vi "_fgv_sessions.vi"(7 "Operation":T7=enum."GetData", 8 "error in":errorcluster caption="error in (no error)", 10 "Session User Data in (None)":T1={"IDN string"="", "Instrument FW"="", "Instr type"="", "Instr type for err. msg."="", "Installed Options"=[], "Ignore Error Messages"="", "Logging params"=variant, "OPC Timeout"=5000, "VISA Timeout"=10000, "STB Poll VISA Timeout"=5000, "Additional Flags"=4, "Wait Before Read"=0, "Wait Before Write"=0, "Option String Flags"=0, "IO Segment Size"=10000000, "VISA Access Mode"=4, "Interface Type"=enum."TCPIP", "OPC Wait Mode"=enum."STBpolling", "Bin Float Number  Format"=enum."Float_4_Bytes_Swapped", "Bin Integer Number Format"=enum."Int32_4_Bytes_Swapped", "Simulate"=FALSE, "VXIcapable"=TRUE, "Duplicate Session"=FALSE, "Add LF to Write"=TRUE, "Logging"=FALSE, "Fast Sweep"=FALSE, "Query Instrument Status"=TRUE, "Check Range"=TRUE, "Check Options"=TRUE} {"VISA Access Mode" items=["VISA Defaults"=0, "Exclusive Lock"=1, "Load Settings"=4]; "IO Segment Size" format="%#.6p"; "Additional Flags" format="%011b"}, 11 "VISA resource name":refnum<visa-resource-name>) -> (0 "error out":errorcluster, 1 "Session Ix out":i32, 2 "Session User Data out":T1={"IDN string"="", "Instrument FW"="", "Instr type"="", "Instr type for err. msg."="", "Installed Options"=[], "Ignore Error Messages"="", "Logging params"=variant, "OPC Timeout"=5000, "VISA Timeout"=10000, "STB Poll VISA Timeout"=5000, "Additional Flags"=4, "Wait Before Read"=0, "Wait Before Write"=0, "Option String Flags"=0, "IO Segment Size"=10000000, "VISA Access Mode"=4, "Interface Type"=enum."TCPIP", "OPC Wait Mode"=enum."STBpolling", "Bin Float Number  Format"=enum."Float_4_Bytes_Swapped", "Bin Integer Number Format"=enum."Int32_4_Bytes_Swapped", "Simulate"=FALSE, "VXIcapable"=TRUE, "Duplicate Session"=FALSE, "Add LF to Write"=TRUE, "Logging"=FALSE, "Fast Sweep"=FALSE, "Query Instrument Status"=TRUE, "Check Range"=TRUE, "Check Options"=TRUE} {"VISA Access Mode" items=["VISA Defaults"=0, "Exclusive Lock"=1, "Load Settings"=4]; "IO Segment Size" format="%#.6p"; "Additional Flags" format="%011b"}, 3 "VISA resource name out":refnum<visa-resource-name>)   [LabVIEW 2022 SP3, in "hmp4000_rsidr_core.lvlib"]
uses:
  hmp4000_rsidr_core.lvlib
  _type_Operation_Fgv_Session.ctl
  type_Session_Data.ctl
  type_VisaAccessMode.ctl
  type_InterfaceType.ctl
  type_OPC_Wait_Mode.ctl
  type_Binary_Float_Number_Format.ctl
  type_Binary_Integer_Number_Format.ctl
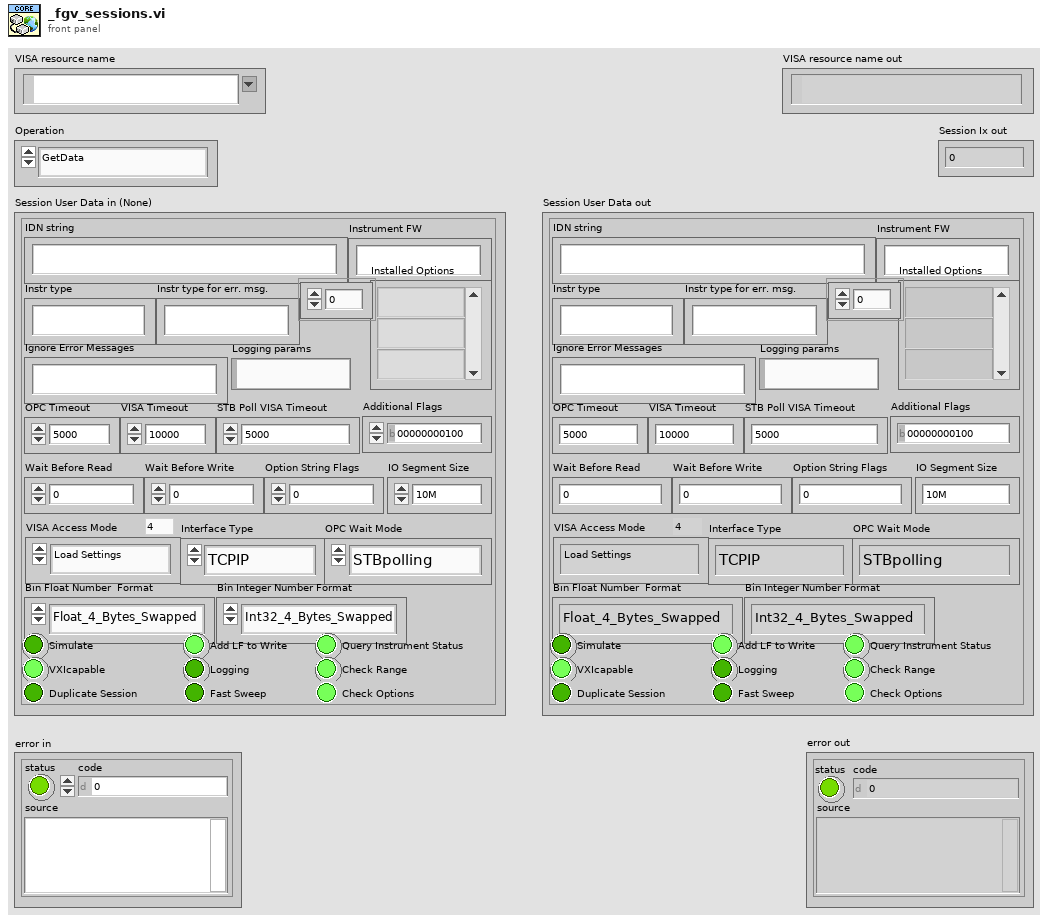
[diagram p1: front panel]
types:
  T1 = typedef "hmp4000_rsidr_core.lvlib/type_Session_Data.ctl" = cluster{"IDN string":string, "Instrument FW":string, "Instr type":string, "Instr type for err. msg.":string, "Installed Options":string[], "Ignore Error Messages":string, "Logging params":variant, "OPC Timeout":i32, "VISA Timeout":i32, "STB Poll VISA Timeout":i32, "Additional Flags":i32, "Wait Before Read":i32, "Wait Before Write":i32, "Option String Flags":i32, "IO Segment Size":i64, "VISA Access Mode":T2, "Interface Type":T3, "OPC Wait Mode":T4, "Bin Float Number  Format":T5, "Bin Integer Number Format":T6, "Simulate":bool, "VXIcapable":bool, "Duplicate Session":bool, "Add LF to Write":bool, "Logging":bool, "Fast Sweep":bool, "Query Instrument Status":bool, "Check Range":bool, "Check Options":bool}
  T2 = typedef "hmp4000_rsidr_core.lvlib/type_VisaAccessMode.ctl" = u16
  T3 = typedef "hmp4000_rsidr_core.lvlib/type_InterfaceType.ctl" = enum16{"Unknown", "GPIB", "VXI", "GPIB_VXI", "ASRL", "PXI", "TCPIP", "USB", "SOCKET"}
  T4 = typedef "hmp4000_rsidr_core.lvlib/type_OPC_Wait_Mode.ctl" = enum16{"STBpolling", "STBpollingSlow", "STBpollingSuperSlow", "ServiceRequest", "OPCquery"}
  T5 = typedef "hmp4000_rsidr_core.lvlib/type_Binary_Float_Number_Format.ctl" = enum16{"Float_4_Bytes_Swapped", "Float_4_Bytes", "Double_8_Bytes_Swapped", "Double_8_Bytes"}
  T6 = typedef "hmp4000_rsidr_core.lvlib/type_Binary_Integer_Number_Format.ctl" = enum16{"Int32_4_Bytes_Swapped", "Int32_4 Bytes", "Int16_2_Bytes_Swapped", "Int16_2_Bytes"}
  T7 = typedef "hmp4000_rsidr_core.lvlib/_type_Operation_Fgv_Session.ctl" = enum16{"Initialize", "GetData", "SetData", "Clear", "GetSessionIx"}
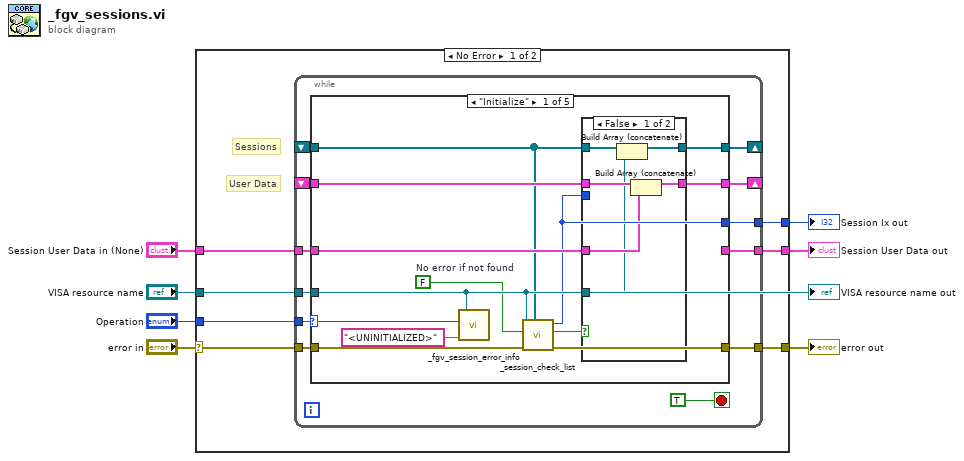
[diagram p0: block diagram]
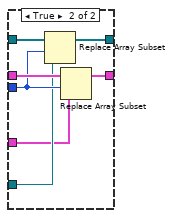
[diagram p2: hidden frame]
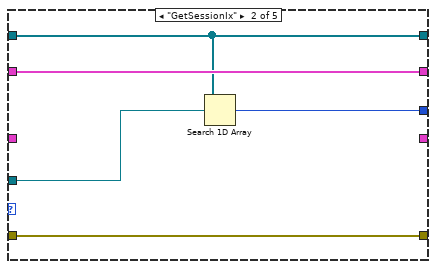
[diagram p3: hidden frame]
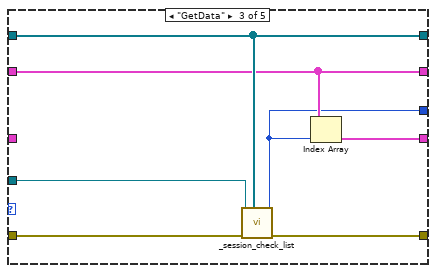
[diagram p4: hidden frame]
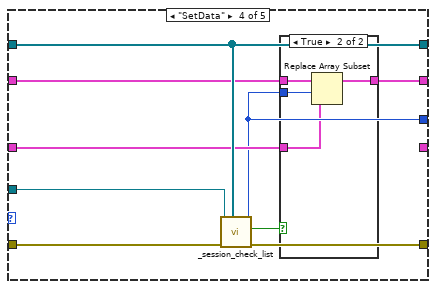
[diagram p5: hidden frame]
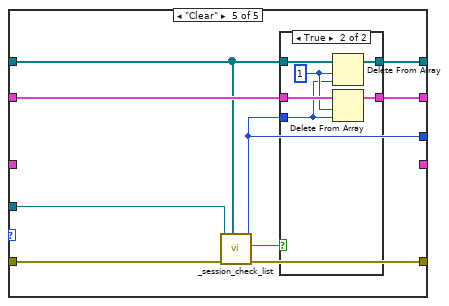
[diagram p7: hidden frame]
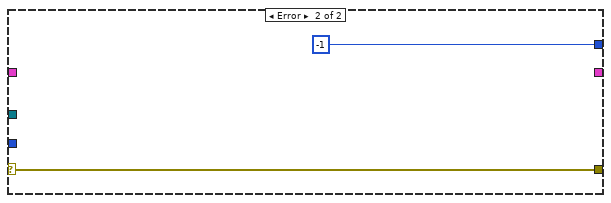
[diagram p9: hidden frame]
diagram:
  n1 = case shown="No Error" "error in" {
    selector: "error in" -> [w13 w97]
    tunnel: "Operation" -> [w10 _]
    tunnel: "Session User Data in (None)" -> [w11 _]
    tunnel: "VISA resource name" -> [w9 _]
    tunnel: [w14 _] -> w6
    tunnel: [w12 w97] -> w2
    tunnel: [w8 -1 ("Session list index out")] -> w1
    frame No Error {
      # "User Data"
      # "Sessions"
      n2 = while {
        tunnel: [w16] -> w14
        tunnel: w13 -> [w19]
        tunnel: [w26] -> w12
        tunnel: w11 -> [w25]
        tunnel: w10 -> [w24]
        tunnel: w9 -> [w23]
        shift-right: [w21] -> _
        shift-left: _ -> [w22]
        shift-right: [w17] -> _
        shift-left: _ -> [w18]
        tunnel: [w15] -> w8
        stop <- TRUE stop-if-true
        n3 = case "Operation case" shown="\"Initialize\"" w24 {
          selector: w24 -> [w27 _ _ _ _]
          tunnel: w23 -> [w30 w54 w62 w72 w86]
          tunnel: w19 -> [w39 w57 w64 w73 w87]
          tunnel: [w38 w57 w63 w67 w85] -> w26
          tunnel: w22 -> [w33 w55 w61 w71 w81]
          tunnel: w25 -> [w34 _ _ w69 _]
          tunnel: [w32 w55 w61 w71 w80] -> w21
          tunnel: w18 -> [w35 w56 w59 w70 w84]
          tunnel: [w31 w56 w59 w68 w82] -> w17
          tunnel: [_ _ w60 _ _] -> w16
          tunnel: [w28 w53 w58 w65 w79] -> w15
          frame "Initialize" {
            w37 = FALSE  # No error if not found
            n4 = call "_fgv_session_error_info.vi"("Session Error Info in (\"\")"="<UNINITIALIZED>" ("Session Error Info in (\"\")"), "Operation"=w27, "Session in"=w30) -> ()  [unwired: 3 in, 2 out]
            n5 = call "_session_check_list.vi"("VISA resource names in"=w33, "error in"=w39, "Error if not found (T)"=w37, "VISA resource name"=w30) -> ("error out"=w38:errorcluster, "Found in the list"=w36:bool, "Session list index out"=w28:i32)  [unwired: 5 in]
            n6 = case shown="False" w36 {
              tunnel: w35 -> [w43 w52]
              tunnel: w34 -> [w42 w46]
              tunnel: w28 -> [_ w48]
              tunnel: w30 -> [w41 w47]
              tunnel: w33 -> [w45 w50]
              tunnel: [w44 w49] -> w32
              tunnel: [w40 w51] -> w31
              frame False {
                n7 = Build Array (concatenate)(w45, w41) -> (w44:refnum<visa-resource-name>[])
                n8 = Build Array (concatenate)(w43, w42) -> (w40:T1[])
              }
              frame True {
                n9 = Replace Array Subset(array=w50, new element=w47, index=w48) -> (w49:refnum<visa-resource-name>[])
                n10 = Replace Array Subset(array=w52, new element=w46, index=w48) -> (w51:T1[])
              }
            }
          }
          frame "GetSessionIx" {
            n11 = Search 1D Array(1D array=w55, element=w54) -> (index of element=w53:i32)  [unwired: 1 in]
          }
          frame "GetData" {
            n12 = call "_session_check_list.vi"("VISA resource names in"=w61, "error in"=w64, "VISA resource name"=w62) -> ("error out"=w63:errorcluster, "Session list index out"=w58:i32)  [unwired: 6 in, 1 out]
            n13 = Index Array(array=w59, index=w58) -> (element=w60:T1)
          }
          frame "SetData" {
            n14 = call "_session_check_list.vi"("VISA resource names in"=w71, "error in"=w73, "VISA resource name"=w72) -> ("error out"=w67:errorcluster, "Found in the list"=w66:bool, "Session list index out"=w65:i32)  [unwired: 6 in]
            n15 = case shown="True" w66 {
              tunnel: w70 -> [w74 w78]
              tunnel: w69 -> [_ w75]
              tunnel: [w74 w77] -> w68
              tunnel: w65 -> [_ w76]
              frame False {
              }
              frame True {
                n16 = Replace Array Subset(array=w78, new element=w75, index=w76) -> (w77:T1[])
              }
            }
          }
          frame "Clear" {
            n17 = call "_session_check_list.vi"("VISA resource names in"=w81, "error in"=w87, "VISA resource name"=w86) -> ("error out"=w85:errorcluster, "Found in the list"=w83:bool, "Session list index out"=w79:i32)  [unwired: 6 in]
            n18 = case shown="True" w83 {
              tunnel: w84 -> [w89 w93]
              tunnel: w79 -> [_ w90]
              tunnel: [w89 w92] -> w82
              tunnel: w81 -> [w88 w95]
              tunnel: [w88 w94] -> w80
              frame False {
              }
              frame True {
                w91 = 1 ("length")
                n19 = Delete From Array(array=w95, length=w91, index=w90) -> (array with subset deleted=w94:refnum<visa-resource-name>[])  [unwired: 1 out]
                n20 = Delete From Array(array=w93, length=w91, index=w90) -> (array with subset deleted=w92:T1[])  [unwired: 1 out]
              }
            }
          }
        }
      }
    }
    frame Error {
    }
  }
  "error out" <- w2
  "Session User Data out" <- w6
  "Session Ix out" <- w1
  "VISA resource name out" <- "VISA resource name"
